vi "Get NATS Connection.vi"(8 "error in":errorcluster {"code" format="Error %.0f"}, 11 "NATS Client.lvlib:NATS Client.lvclass":refnum<class "NATS Client.lvclass">) -> (0 "error out":errorcluster, 3 "NATS Connection":T1={"connection ID"=refnum, "server INFO"="", "timeout ms"=5000, "verbose?"=FALSE, "server headers?"=FALSE, "client headers?"=FALSE})   [LabVIEW 2024, in "NATS Client.lvlib" / "NATS Client.lvclass"]
uses:
  NATS Client.lvclass
  <vilib>/NATS/NATS Core/Controls/nats connection.ctl
  NATS Client.lvclass/NATS Client.ctl
  <vilib>/NATS/NATS Core/NATS Core.lvlib
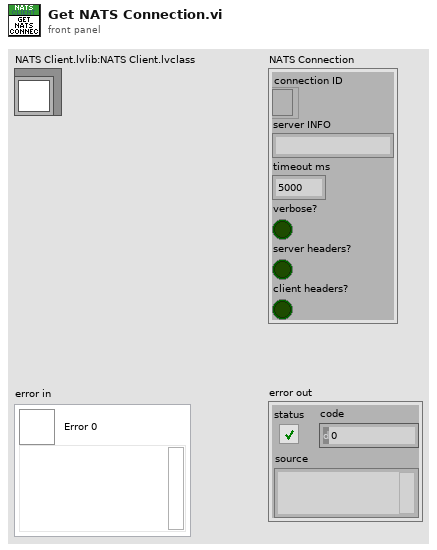
[diagram p1: front panel]
types:
  T1 = typedef "NATS Core.lvlib/nats connection.ctl" = cluster{"connection ID":refnum<k5>, "server INFO":string, "timeout ms":i32, "verbose?":bool, "server headers?":bool, "client headers?":bool}
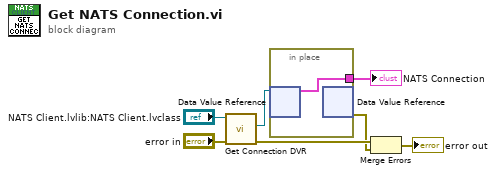
[diagram p0: block diagram]
diagram:
  n1 = call "Get Connection DVR.vi"("error in"="error in", "NATS Client in"="NATS Client.lvlib:NATS Client.lvclass") -> ("error out"=w4:errorcluster, "NATS Connection"=w5:refnum<data-value>)  [unwired: 7 in, 1 out]
  n2 = in-place {
    in-place-border: [w8] -> w6
    n3 = in-place-dvr #1 ("Data Value Reference Read / Write Element")(w5) -> (w8:T1)  [unwired: 1 out]
    n4 = in-place-dvr #1() -> (w2:errorcluster)  [unwired: 1 in, 1 out]
  }
  "NATS Connection" <- w6
  n5 = Merge Errors(w4, w2) -> (→"error out":errorcluster)
